vi "Create Pattern Script - Rd Data Frame.vi"(8 "error in (no error)":errorcluster, 10 "FRM Data":T1 {"Addr" format="%x"; "Data" format="%x"}, 11 "SPI Root Pattern Creator in":refnum<class "SPI Root Pattern Creator.lvclass">) -> (0 "error out":errorcluster, 2 "String":string, 3 "SPI Root Pattern Creator out":refnum<class "SPI Root Pattern Creator.lvclass">)   [LabVIEW 2018, in "SPI Root Pattern Creator.lvlib" / "SPI Root Pattern Creator.lvclass"]
uses:
  SPI Root Pattern Creator.lvclass
  Ctls/Frame Data - SPI_3W.ctl
  Ctls/RW Options.ctl
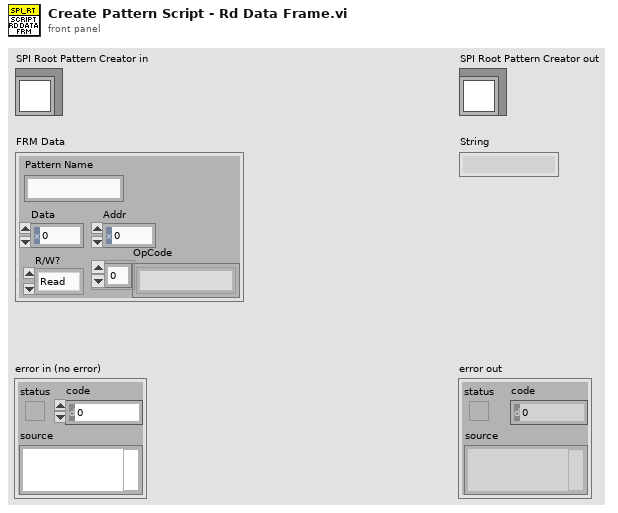
[diagram p1: front panel]
types:
  T1 = typedef "Frame Data - SPI_3W.ctl" = cluster{"Pattern Name":string, "Data":u16, "Addr":u16, "OpCode":string[], "R/W?":T2}
  T2 = typedef "RW Options.ctl" = enum16{"Read", "Write", "R/W"}
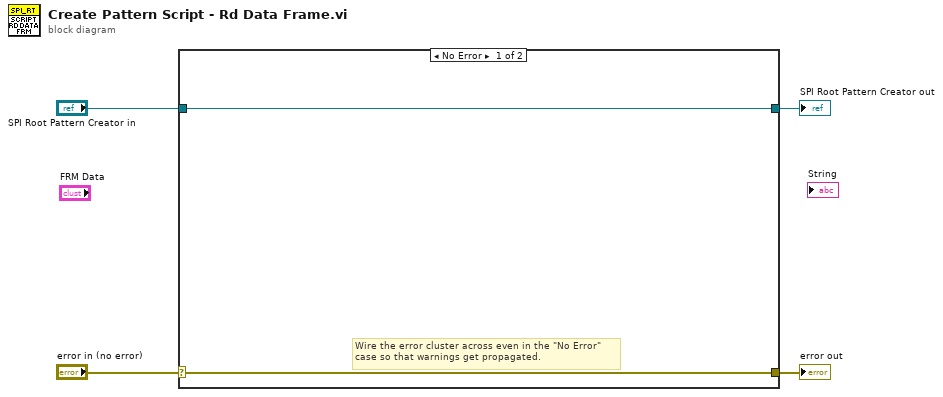
[diagram p0: block diagram]
diagram:
  n1 = case shown="No Error" "error in (no error)" {
    selector: "error in (no error)" -> [w5 w8]
    tunnel: [w5 w8] -> w3
    tunnel: [w6 w7] -> w1
    tunnel: "SPI Root Pattern Creator in" -> [w6 w7]
    frame No Error {
      # "Wire the error cluster across even in the \"No Error\"\ncase so that warnings get propagated."
    }
    frame Error {
    }
  }
  "error out" <- w3
  "SPI Root Pattern Creator out" <- w1
